vi "Dead Zone.vi"(10 "Dead Zone":dbl=0.2, 11 "Input":dbl) -> (3 "Output":dbl)   [LabVIEW 2012]
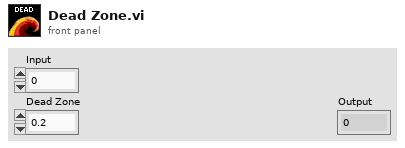
[diagram p1: front panel]
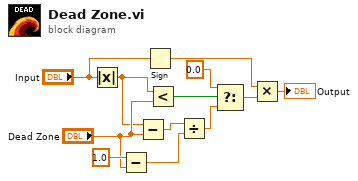
[diagram p0: block diagram]
diagram:
  n1 = Absolute Value(x="Input") -> (abs(x)=w1:dbl)
  n2 = Subtract(x=1.0, y="Dead Zone") -> (x-y=w6:dbl)
  n3 = Subtract(x=w1, y="Dead Zone") -> (x-y=w10:dbl)
  n4 = Sign(1:"Input") -> (0:w2:dbl)
  n5 = Less?(x=w1, y="Dead Zone") -> (x < y?=w12:bool)
  n6 = Divide(x=w10, y=w6) -> (x/y=w9:dbl)
  n7 = Select(t=0.0, s=w12, f=w9) -> (s? t:f=w4:dbl)
  n8 = Multiply(x=w2, y=w4) -> (x*y=→"Output":dbl)
